vi "pH buffer.vi"(2 "pH error":dbl=0.75 format="%.2f", 3 "Temperature":dbl=0.5 format="%.2f", 4 "V/T":dbl format="%.5f", 5 "pH scale in":T1 {"Buffers"."V/T" format="%.5f"; "Buffers"."Buffer" format="%.2f"; "Temperature" format="%.2f"}) -> (0 "Theoretical pH":dbl format="%.2f", 1 "pH scale out":T1 {"Buffers"."V/T" format="%.5f"; "Buffers"."Buffer" format="%.2f"; "Temperature" format="%.2f"})   [LabVIEW 2012]
uses:
  pH scale.ctl
panel:
  # "C"
  # "C"
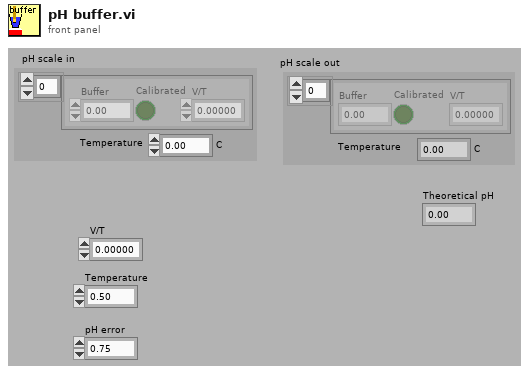
[diagram p1: front panel]
types:
  T1 = typedef "pH scale.ctl" = cluster{"Buffers":cluster{"Buffer":dbl, "Calibrated":bool, "V/T":dbl}[], "Temperature":dbl}
  T2 = cluster{"Buffer":dbl, "Calibrated":bool, "V/T":dbl}[]
  T3 = cluster{"Buffer":dbl, "Calibrated":bool, "V/T":dbl}
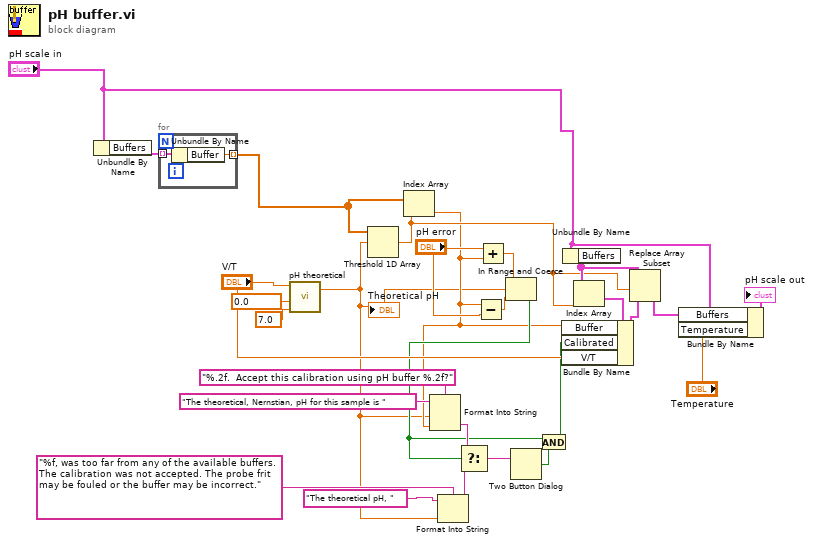
[diagram p0: block diagram]
diagram:
  n1 = Unbundle By Name("pH scale in") -> ("Buffers"=w19:T2)
  n2 = for {
    tunnel: w19 -> [w30] mode=indexing
    tunnel: [w29] -> w2 mode=indexing
    n3 = Unbundle By Name(w30) -> ("Buffer"=w29:dbl)
  }
  n4 = call "pH theoretical.vi"("pH cal"=7.0, "V/T cal"=0.0, "V/T"="V/T") -> ("Theoretical pH"=w3:dbl)  [unwired: 2 in]
  n5 = Threshold 1D Array(2:w3, 3:w2) -> (0:w21:dbl)  [unwired: 1 in]
  n6 = Index Array(array=w2, index=w21) -> (element=w4:dbl)
  n7 = Format Into String(format string="%.2f.  Accept this calibration using pH buffer %.2f?" ("Format String"), initial string="The theoretical, Nernstian, pH for this sample is " ("message"), w3, w4) -> (resulting string=w12:string)  [unwired: 1 in, 1 out]
  n8 = Format Into String(format string="%f, was too far from any of the available buffers. The calibration was not accepted. The probe frit may be fouled or the buffer may be incorrect." ("Format String"), initial string="The theoretical pH, " ("f"), w3) -> (resulting string=w5:string)  [unwired: 1 in, 1 out]
  n9 = Subtract(x=w4, y="pH error") -> (x-y=w25:dbl)
  n10 = Add(x="pH error", y=w4) -> (x+y=w26:dbl)
  n11 = In Range and Coerce(upper limit=w26, x=w3, lower limit=w25) -> (In Range?=w9:bool)  [unwired: 1 out]
  n12 = Select(t=w12, s=w9, f=w5) -> (s? t:f=w11:string)
  n13 = Two Button Dialog(message=w11) -> (T button?=w10:bool)  [unwired: 2 in]
  n14 = And(x=w9, y=w10) -> (x .and. y?=w8:bool)
  n15 = Unbundle By Name("pH scale in") -> ("Buffers"=w23:T2)
  n16 = Index Array(array=w23, index=w21) -> (element=w24:T3)
  n17 = Bundle By Name(cluster=w24, "Buffer"=w4, "Calibrated"=w8, "V/T"="V/T") -> (w22:T3)
  n18 = Replace Array Subset(array=w23, new element=w22, index=w21) -> (w20:T2)
  n19 = Bundle By Name(cluster="pH scale in", "Buffers"=w20, "Temperature"="Temperature") -> (→"pH scale out":T1)
